vi "SENS_COUP_PAR_STAT.vi"(0 "VISA IN":refnum<visa-resource-name>, 1 "Time Domain Trace Coupling ON/OFF":bool, 5 "error in":errorcluster, 7 "Channel":i32) -> (14 "VISA Out":refnum<visa-resource-name>, 19 "error out":errorcluster)   [LabVIEW 2018, in "PNA-X.lvlib"]
doc: "SENSe<cnum>:COUPle:PARameter[:STATe] <bool> \n1733\n\n(Read-Write) Turns ON and OFF Time Domain Trace Coupling. All of the measurements in the \nspecified channel are coupled. \nTo select Transform parameters to couple, use CALC:TRAN:COUP:PAR \nTo select Gating parameters to couple, use CALC:FILT:COUP:PAR \nLearn more about Time Domain Trace Coupling. \nParameters \n<cnum> Any existing channel number; if unspecified, value is set to 1. \n<bool> ON (or 1) - Turns ON Time Domain Trace Coupling. \nOFF (or 0) - Turns OFF Time Domain Trace Coupling. \nExamples SENS:COUP:PAR 0 \nsense2:couple:parameter:state on \nQuery Syntax SENSe<cnum>:COUPle:PARameter[:STATe]? \nReturn Type Boolean \nDefault ON (or 1) \n1734\n\nSense:FOM (Frequency Offset) Commands \nControls the frequency offset settings which cause stimulus and response frequencies to be different. \nNote: These commands supersede previous FOM commands. Although the old commands will continue to work, \nthey can NOT be mixed with these new commands. \nClick on a blue keyword to view the command details. \nSee Also \nExample Programs \nLearn about Frequency Offset \nSynchronizing the PNA and Controller \nSCPI Command Tree"
uses:
  PNA-X.lvlib
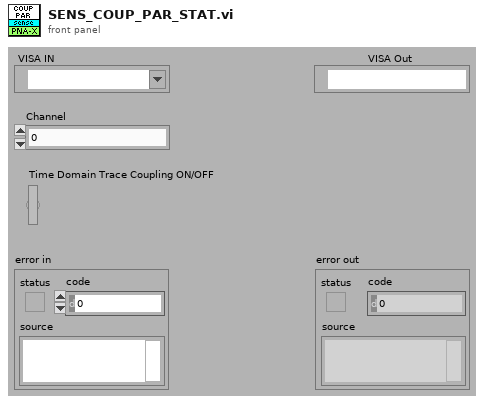
[diagram p1: front panel]
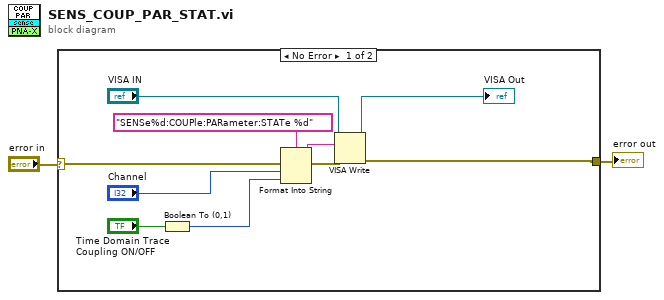
[diagram p0: block diagram]
diagram:
  n1 = case shown="No Error" "error in" {
    selector: "error in" -> [w12 w13]
    tunnel: [w7 w13] -> w1
    frame No Error {
      n2 = Boolean To (0,1)(Boolean="Time Domain Trace Coupling ON/OFF") -> (0, 1=w3:i16)
      n3 = Format Into String(format string="SENSe%d:COUPle:PARameter:STATe %d" ("Cmdline"), error in=w12, "Channel", w3) -> (resulting string=w10:string, error out=w11:errorcluster)  [unwired: 1 in]
      n4 = VISA Write(VISA resource name="VISA IN", write buffer=w10, error in (no error)=w11) -> (VISA resource name out=→"VISA Out":refnum<visa-resource-name>, error out=w7:errorcluster)  [unwired: 1 out]
    }
    frame Error {
    }
  }
  "error out" <- w1
